vi "ADC Initiate Digitizing Process.vi"(8 "error in":errorcluster, 10 "Is first multiplex cycle? (True)":bool=TRUE, 11 "adc session in":T1={"niScope"={"channel cfg"=[], "sessions"=[], "multi cards"=FALSE, "channels"=0, "type"=enum."n/a", "memory [B/chn]"=0, "ext. clock [Hz]"=0.0, "samples count"=0, "use streaming"=FALSE, "proc setup"={"packet size [smpl]"=0, "current timeout [s]"=0.0, "blk2blk timeout [s]"=0.0, "event time"=timestamp(0 s since 1904-01-01), "temp sampl T [s]"=0.0, "data queue"=refnum, "stop notifier"=refnum, "proc ref"=refnum}, "sample width [B]"=0, "ranges [V]"=[], "trigger setup"={"coupling"=1, "level [V]"=0.0, "slope"=0, "mode"=enum."Immediate", "pre-trigger [%]"=0.0}, "fs [Hz]"=0.0, "bitres [bit]"=0, "clock source"=enum."VAL_NO_SOURCE"}, "3458A"={"channels"=[], "sync unit"={"VISA"="", "type"=enum."Picotest U6200A"}, "awg unit"={"type"=enum."Agilent 331xxA to 332xxA", "VISA"="", "enable 10MHz ref"=FALSE, "cmi ckd2"={"VISA"="", "clock source"=enum."Auto", "manual ref clk"=FALSE, "ref clock [Hz]"=0.0, "div mode"=enum."Set divisor directly"}, "cmi sync v3"={"VISA"="", "baud rate [bd/s]"=115200, "source"=enum."Auto", "hv range"=enum."1kV", "fsrc is fixed"=FALSE, "fsrc [Hz]"=10000000.0, "freq integ [s]"=1.0, "freq filter"=5, "trig level"=enum."TTL 5V", "chn1 mode"=enum."Source divider", "chn1 level"=enum."Positive 5V", "chn2 mode"=enum."Source divider", "chn2 level"=enum."Positive 5V", "chn2 div"=1, "chn3 mode"=enum."Chn 1 Active", "chn3 level"=enum."Positive 5V", "chn1 div entry"=enum."Calculate nearest divisor from measured fx", "chn1 dev limit [%]"=1.0, "chn1 check dev"=FALSE}, "trigger"={"source"=enum."Immediate", "slope"=enum."POS", "coupling"=enum."DC", "level [V]"=0.0, "hysteresis [V]"=0.0, "pre-trigger [%]"=0.0}, "HMF2500 cfg"={"Baud Rate"=9600, "Parity"=0, "Data Bits"=8, "Flow Control"=4}}, "sync mode"=enum."MASTER-SLAVE, MASTER clocked by TIMER", "streaming mode"=FALSE, "idn mode"=enum."Auto", "sampling mode"=enum."DCV", "sample memory [B]"=0, "proc setup"={"channel id"=0, "packet size [smpl]"=0, "current timeout [s]"=0.0, "blk2blk timeout [s]"=0.0, "event time"=timestamp(0 s since 1904-01-01), "stop notifier"=refnum, "data queues"=[], "proc refs"=[], "bus semaphore"=refnum}, "sample size [B]"=0, "sample count"=0, "aux data"={"channel id"=0, "valid?"=[], "gain [V]"=[], "timestamp [s]"=[], "Ts [s]"=0.0, "abs timestamp"=timestamp(0 s since 1904-01-01), "t [deg C]"=[], "multiplex timestamp [s]"=-1.0, "only multiplex?"=FALSE, "multiplex smpl offset"=0, "overflow?"=FALSE}, "ranges [V]"=[], "aperture [s]"=0.0, "LEVEL trigger"={"edge"=enum."POS", "level [V]"=0.0, "coupling"=enum."DC"}, "trigger mode"=enum."AUTO", "measure temp.?"=FALSE, "disp mesages"=[], "shared bus?"=FALSE, "disable display?"=FALSE, "aper mode"=enum."Manual", "aper rules"=[], "multiplex"={"cycles"=0, "delay [s]"=0.0, "enabled"=FALSE, "overhead [s]"=1.0, "tot smpls"=0, "sub-rec"=0, "overhead [%]"=0.0, "emulated"=FALSE}, "F8588 lpf"=enum."Off", "F8588 pll"=enum."Off", "F8588 couple"=enum."DC, auto", "fs"={"freq mode"=enum."fs or Ts", "fs [Hz]"=0.0, "fref [Hz]"=0.0, "mul"=0.0, "div"=0.0}, "fs mode"=enum."fs or Ts"}, "dsdll"={"dsdll"={"dsdll path"=path "", "dsdll handle"=[], "output devices"=[], "capture devices"=[]}, "channels"=0, "device id"=0, "channel idns"=[], "proc setup"={"packet size [smpl]"=0, "current timeout [s]"=0.0, "blk2blk timeout [s]"=0.0, "event time"=timestamp(0 s since 1904-01-01), "data queue"=refnum, "stop notifier"=refnum, "proc ref"=refnum}, "samples count"=0, "fs [Hz]"=0.0}, "type"=enum."niScope", "channel idn str"=[], "aux instr idn str"=[], "modified?"=FALSE, "simadc"={"channels"=[], "range [V]"=0.0, "Ts step [s]"=0.0, "time [s]"=0.0, "fs [Hz]"=0.0, "count"=0, "smpl offset"=0, "set count"=0, "bit res"=0}, "force rst?"=FALSE, "exit mode"=enum."Immediate reset", "exit dly"=0.0, "exit tmr"=timestamp(0 s since 1904-01-01), "busy?"=FALSE, "accessed?"=FALSE, "multiplex"={"Type"=enum."Dummy", "gen com ssn"={"visa"="", "primary"=enum."None", "secondary"=enum."None", "channels"=[]}, "delay before [s]"=0.0, "delay post [s]"=0.0, "sequence"=[], "enabled"=FALSE, "ref timestamp [s]"=0.0, "idn string"="", "dev niScope"="", "niScope idx"=0, "QPMX ssn"={"visa"="", "switch mode"=enum."Switched by TWM", "sequence"=[], "timing delays"=[], "polarity"=enum."Positive", "ss delay (s)"=2.0, "internal timer (s)"=1.0, "Last loaded sequence file"=path "", "startup delay (s)"=2.0}, "VISA mux ssn"={"VISA"="", "paths"=[], "idn command"="", "serial cfg"={"Baud rate"=9600, "Data bits"=8, "Parity"=0, "Stop bits"=10, "Flow control"=0, "End Mode Read"=enum."None", "End Mode Write"=enum."None", "Term character"=0, "Term enable"=FALSE}}}, "keysight dso"={"VISA"="", "channels"=[], "bw limit [Hz]"=0.0, "resolution"=enum."Basic", "trig noise reject"=enum."Normal", "N"=0, "trigger config"={"trigger source"=enum."Immediate", "trigger slope"=enum."Negative", "level [V]"=0.0, "hysteresis [V]"=0.001, "pre-trig [%]"=50}, "fs [Hz]"=0.0, "timeout stop"=timestamp(0 s since 1904-01-01), "waiting for opc"=FALSE, "fetch offset [smpl]"=0, "abs timestamp"=timestamp(0 s since 1904-01-01), "ranges [V]"=[], "decimation"=1.0, "ext ref"=FALSE, "emulate aperture"=FALSE, "model"=enum."DSO91304"}, "cdaq"={"mclk [Hz]"=12800000.0, "ADC task"="", "mclk reference"="", "fs [Hz]"=50000.0, "queue adc cmd"=refnum, "queue adc data"=refnum, "adc proc ref"=refnum, "channels"=[], "last channels"=[], "timeout"=timestamp(0 s since 1904-01-01), "N"=1000, "mclk mode"=enum."Free running", "ext mclk source"=""}, "ignore overload"=FALSE, "ADS127L21"={"VISA"="", "chn list"=[], "record size"=0, "phys. channels"=0, "adc fifo size"=0, "channels"=[], "ext refclk?"=FALSE, "fs [Hz]"=0.0, "ext refclk [Hz]"=0.0, "meas refclk [Hz]"=0.0, "EXTOUT mode"=enum."ADCCLK", "EXTOUT polarity"=enum."NORM", "EXTOUT divisor"=0}} {"ADS127L21"."channels"."Channel" min=1 max=8 step=1; "cdaq"."last channels"."Channel id" min=0 step=1; "cdaq"."channels"."Channel id" min=0 step=1; "keysight dso"."decimation" min=1.0; "keysight dso"."bw limit [Hz]" format="%#_6p"; "keysight dso"."channels"."Offset [V]" format="%#_6p"; "keysight dso"."channels"."Range [Vpk]" min=0.0 format="%#_6p"; "keysight dso"."channels"."Channel" min=1; "multiplex"."VISA mux ssn"."serial cfg"."Flow control" items=["None", "XON/XOFF", "CTS/RTS", "XON/XOFF + CTS/RTS", "DTR/DSR", "XON/XOFF + DTR/DSR"]; "multiplex"."VISA mux ssn"."serial cfg"."Stop bits" items=["1 bit"=10, "1.5 bits"=15, "2 bits"=20]; "multiplex"."VISA mux ssn"."serial cfg"."Parity" items=["None", "Odd", "Even", "Mark", "Space"]; "multiplex"."VISA mux ssn"."serial cfg"."Data bits" items=["5 bits"=5, "6 bits"=6, "7 bits"=7, "8 bits"=8]; "multiplex"."VISA mux ssn"."serial cfg"."Baud rate" items=["150 Bd"=150, "300 Bd"=300, "600 Bd"=600, "1200 Bd"=1200, "2400 Bd"=2400, "4800 Bd"=4800, "9600 Bd"=9600, "19.2 kBd"=19200, "38.4 kBd"=38400, "57.6 kBd"=57600, "115.2 kBd"=115200]; "multiplex"."QPMX ssn"."startup delay (s)" min=0.0 step=1.0; "multiplex"."QPMX ssn"."internal timer (s)" min=0.0 step=1.0; "multiplex"."QPMX ssn"."ss delay (s)" min=0.0 step=1.0; "multiplex"."QPMX ssn"."timing delays" min=1 max=255 step=1; "3458A"."awg unit"."HMF2500 cfg"."Flow Control" items=["None", "XON/XOFF", "RTS/CTS", "XON/XOFF & RTS/CTS", "DTR/DSR", "XON/XOFF & DTR/DSR"]; "3458A"."awg unit"."HMF2500 cfg"."Data Bits" items=["7"=7, "8"=8]; "3458A"."awg unit"."HMF2500 cfg"."Parity" items=["None", "Odd", "Even", "Mark", "Space"]; "3458A"."awg unit"."HMF2500 cfg"."Baud Rate" items=["300"=300, "600"=600, "1200"=1200, "2400"=2400, "4800"=4800, "9600"=9600, "19200"=19200]; "3458A"."awg unit"."cmi sync v3"."chn2 div" min=1 max=100000000 step=1; "3458A"."awg unit"."cmi sync v3"."fsrc [Hz]" format="%_8p"; "3458A"."channels"."Range [Vpk]" min=0.0; "niScope"."trigger setup"."pre-trigger [%]" format="%.2f"; "niScope"."trigger setup"."level [V]" format="%.2f"; "niScope"."trigger setup"."coupling" items=["AC"=0, "DC"=1, "HF Reject"=3, "LF Reject"=4, "AC Plus HF Reject"=1001]; "niScope"."channel cfg"."Range [Vpk]" min=0.0; "niScope"."channel cfg"."Channel" min=0}) -> (0 "error out":errorcluster, 3 "adc session out":T1={"niScope"={"channel cfg"=[], "sessions"=[], "multi cards"=FALSE, "channels"=0, "type"=enum."n/a", "memory [B/chn]"=0, "ext. clock [Hz]"=0.0, "samples count"=0, "use streaming"=FALSE, "proc setup"={"packet size [smpl]"=0, "current timeout [s]"=0.0, "blk2blk timeout [s]"=0.0, "event time"=timestamp(0 s since 1904-01-01), "temp sampl T [s]"=0.0, "data queue"=refnum, "stop notifier"=refnum, "proc ref"=refnum}, "sample width [B]"=0, "ranges [V]"=[], "trigger setup"={"coupling"=1, "level [V]"=0.0, "slope"=0, "mode"=enum."Immediate", "pre-trigger [%]"=0.0}, "fs [Hz]"=0.0, "bitres [bit]"=0, "clock source"=enum."VAL_NO_SOURCE"}, "3458A"={"channels"=[], "sync unit"={"VISA"="", "type"=enum."Picotest U6200A"}, "awg unit"={"type"=enum."Agilent 331xxA to 332xxA", "VISA"="", "enable 10MHz ref"=FALSE, "cmi ckd2"={"VISA"="", "clock source"=enum."Auto", "manual ref clk"=FALSE, "ref clock [Hz]"=0.0, "div mode"=enum."Set divisor directly"}, "cmi sync v3"={"VISA"="", "baud rate [bd/s]"=115200, "source"=enum."Auto", "hv range"=enum."1kV", "fsrc is fixed"=FALSE, "fsrc [Hz]"=10000000.0, "freq integ [s]"=1.0, "freq filter"=5, "trig level"=enum."TTL 5V", "chn1 mode"=enum."Source divider", "chn1 level"=enum."Positive 5V", "chn2 mode"=enum."Source divider", "chn2 level"=enum."Positive 5V", "chn2 div"=1, "chn3 mode"=enum."Chn 1 Active", "chn3 level"=enum."Positive 5V", "chn1 div entry"=enum."Calculate nearest divisor from measured fx", "chn1 dev limit [%]"=1.0, "chn1 check dev"=FALSE}, "trigger"={"source"=enum."Immediate", "slope"=enum."POS", "coupling"=enum."DC", "level [V]"=0.0, "hysteresis [V]"=0.0, "pre-trigger [%]"=0.0}, "HMF2500 cfg"={"Baud Rate"=9600, "Parity"=0, "Data Bits"=8, "Flow Control"=4}}, "sync mode"=enum."MASTER-SLAVE, MASTER clocked by TIMER", "streaming mode"=FALSE, "idn mode"=enum."Auto", "sampling mode"=enum."DCV", "sample memory [B]"=0, "proc setup"={"channel id"=0, "packet size [smpl]"=0, "current timeout [s]"=0.0, "blk2blk timeout [s]"=0.0, "event time"=timestamp(0 s since 1904-01-01), "stop notifier"=refnum, "data queues"=[], "proc refs"=[], "bus semaphore"=refnum}, "sample size [B]"=0, "sample count"=0, "aux data"={"channel id"=0, "valid?"=[], "gain [V]"=[], "timestamp [s]"=[], "Ts [s]"=0.0, "abs timestamp"=timestamp(0 s since 1904-01-01), "t [deg C]"=[], "multiplex timestamp [s]"=-1.0, "only multiplex?"=FALSE, "multiplex smpl offset"=0, "overflow?"=FALSE}, "ranges [V]"=[], "aperture [s]"=0.0, "LEVEL trigger"={"edge"=enum."POS", "level [V]"=0.0, "coupling"=enum."DC"}, "trigger mode"=enum."AUTO", "measure temp.?"=FALSE, "disp mesages"=[], "shared bus?"=FALSE, "disable display?"=FALSE, "aper mode"=enum."Manual", "aper rules"=[], "multiplex"={"cycles"=0, "delay [s]"=0.0, "enabled"=FALSE, "overhead [s]"=1.0, "tot smpls"=0, "sub-rec"=0, "overhead [%]"=0.0, "emulated"=FALSE}, "F8588 lpf"=enum."Off", "F8588 pll"=enum."Off", "F8588 couple"=enum."DC, auto", "fs"={"freq mode"=enum."fs or Ts", "fs [Hz]"=0.0, "fref [Hz]"=0.0, "mul"=0.0, "div"=0.0}, "fs mode"=enum."fs or Ts"}, "dsdll"={"dsdll"={"dsdll path"=path "", "dsdll handle"=[], "output devices"=[], "capture devices"=[]}, "channels"=0, "device id"=0, "channel idns"=[], "proc setup"={"packet size [smpl]"=0, "current timeout [s]"=0.0, "blk2blk timeout [s]"=0.0, "event time"=timestamp(0 s since 1904-01-01), "data queue"=refnum, "stop notifier"=refnum, "proc ref"=refnum}, "samples count"=0, "fs [Hz]"=0.0}, "type"=enum."niScope", "channel idn str"=[], "aux instr idn str"=[], "modified?"=FALSE, "simadc"={"channels"=[], "range [V]"=0.0, "Ts step [s]"=0.0, "time [s]"=0.0, "fs [Hz]"=0.0, "count"=0, "smpl offset"=0, "set count"=0, "bit res"=0}, "force rst?"=FALSE, "exit mode"=enum."Immediate reset", "exit dly"=0.0, "exit tmr"=timestamp(0 s since 1904-01-01), "busy?"=FALSE, "accessed?"=FALSE, "multiplex"={"Type"=enum."Dummy", "gen com ssn"={"visa"="", "primary"=enum."None", "secondary"=enum."None", "channels"=[]}, "delay before [s]"=0.0, "delay post [s]"=0.0, "sequence"=[], "enabled"=FALSE, "ref timestamp [s]"=0.0, "idn string"="", "dev niScope"="", "niScope idx"=0, "QPMX ssn"={"visa"="", "switch mode"=enum."Switched by TWM", "sequence"=[], "timing delays"=[], "polarity"=enum."Positive", "ss delay (s)"=2.0, "internal timer (s)"=1.0, "Last loaded sequence file"=path "", "startup delay (s)"=2.0}, "VISA mux ssn"={"VISA"="", "paths"=[], "idn command"="", "serial cfg"={"Baud rate"=9600, "Data bits"=8, "Parity"=0, "Stop bits"=10, "Flow control"=0, "End Mode Read"=enum."None", "End Mode Write"=enum."None", "Term character"=0, "Term enable"=FALSE}}}, "keysight dso"={"VISA"="", "channels"=[], "bw limit [Hz]"=0.0, "resolution"=enum."Basic", "trig noise reject"=enum."Normal", "N"=0, "trigger config"={"trigger source"=enum."Immediate", "trigger slope"=enum."Negative", "level [V]"=0.0, "hysteresis [V]"=0.001, "pre-trig [%]"=50}, "fs [Hz]"=0.0, "timeout stop"=timestamp(0 s since 1904-01-01), "waiting for opc"=FALSE, "fetch offset [smpl]"=0, "abs timestamp"=timestamp(0 s since 1904-01-01), "ranges [V]"=[], "decimation"=1.0, "ext ref"=FALSE, "emulate aperture"=FALSE, "model"=enum."DSO91304"}, "cdaq"={"mclk [Hz]"=12800000.0, "ADC task"="", "mclk reference"="", "fs [Hz]"=50000.0, "queue adc cmd"=refnum, "queue adc data"=refnum, "adc proc ref"=refnum, "channels"=[], "last channels"=[], "timeout"=timestamp(0 s since 1904-01-01), "N"=1000, "mclk mode"=enum."Free running", "ext mclk source"=""}, "ignore overload"=FALSE, "ADS127L21"={"VISA"="", "chn list"=[], "record size"=0, "phys. channels"=0, "adc fifo size"=0, "channels"=[], "ext refclk?"=FALSE, "fs [Hz]"=0.0, "ext refclk [Hz]"=0.0, "meas refclk [Hz]"=0.0, "EXTOUT mode"=enum."ADCCLK", "EXTOUT polarity"=enum."NORM", "EXTOUT divisor"=0}} {"ADS127L21"."channels"."Channel" min=1 max=8 step=1; "cdaq"."last channels"."Channel id" min=0 step=1; "cdaq"."channels"."Channel id" min=0 step=1; "keysight dso"."decimation" min=1.0; "keysight dso"."bw limit [Hz]" format="%#_6p"; "keysight dso"."channels"."Offset [V]" format="%#_6p"; "keysight dso"."channels"."Range [Vpk]" min=0.0 format="%#_6p"; "keysight dso"."channels"."Channel" min=1; "multiplex"."VISA mux ssn"."serial cfg"."Flow control" items=["None", "XON/XOFF", "CTS/RTS", "XON/XOFF + CTS/RTS", "DTR/DSR", "XON/XOFF + DTR/DSR"]; "multiplex"."VISA mux ssn"."serial cfg"."Stop bits" items=["1 bit"=10, "1.5 bits"=15, "2 bits"=20]; "multiplex"."VISA mux ssn"."serial cfg"."Parity" items=["None", "Odd", "Even", "Mark", "Space"]; "multiplex"."VISA mux ssn"."serial cfg"."Data bits" items=["5 bits"=5, "6 bits"=6, "7 bits"=7, "8 bits"=8]; "multiplex"."VISA mux ssn"."serial cfg"."Baud rate" items=["150 Bd"=150, "300 Bd"=300, "600 Bd"=600, "1200 Bd"=1200, "2400 Bd"=2400, "4800 Bd"=4800, "9600 Bd"=9600, "19.2 kBd"=19200, "38.4 kBd"=38400, "57.6 kBd"=57600, "115.2 kBd"=115200]; "multiplex"."QPMX ssn"."startup delay (s)" min=0.0 step=1.0; "multiplex"."QPMX ssn"."internal timer (s)" min=0.0 step=1.0; "multiplex"."QPMX ssn"."ss delay (s)" min=0.0 step=1.0; "multiplex"."QPMX ssn"."timing delays" min=1 max=255 step=1; "3458A"."awg unit"."HMF2500 cfg"."Flow Control" items=["None", "XON/XOFF", "RTS/CTS", "XON/XOFF & RTS/CTS", "DTR/DSR", "XON/XOFF & DTR/DSR"]; "3458A"."awg unit"."HMF2500 cfg"."Data Bits" items=["7"=7, "8"=8]; "3458A"."awg unit"."HMF2500 cfg"."Parity" items=["None", "Odd", "Even", "Mark", "Space"]; "3458A"."awg unit"."HMF2500 cfg"."Baud Rate" items=["300"=300, "600"=600, "1200"=1200, "2400"=2400, "4800"=4800, "9600"=9600, "19200"=19200]; "3458A"."awg unit"."cmi sync v3"."chn2 div" min=1 max=100000000 step=1; "3458A"."awg unit"."cmi sync v3"."fsrc [Hz]" format="%_8p"; "3458A"."channels"."Range [Vpk]" min=0.0; "niScope"."trigger setup"."pre-trigger [%]" format="%.2f"; "niScope"."trigger setup"."level [V]" format="%.2f"; "niScope"."trigger setup"."coupling" items=["AC"=0, "DC"=1, "HF Reject"=3, "LF Reject"=4, "AC Plus HF Reject"=1001]; "niScope"."channel cfg"."Range [Vpk]" min=0.0; "niScope"."channel cfg"."Channel" min=0})   [LabVIEW 2020]
doc: "Initiates digitizing process. It starts background processes that starts sampling as soon as trigger condition it meet. Then they either stores samples to the instruments memory and reading them afterwards or streams the data directly. In both cases the sample data are sent to data queue(s). The content of the queue must be read and processed as fast as possible to prevent overflow error so this VI call must be immediatelly followed by fetch loop with 'Fetch From Digitizing Process' function. When fetching is done for whatever reason user must call 'Clenup Digitizing Process' to kill and cleanup all objects related to the digitizing process. It must be called even in case of error.\nVI modifies session content so do not assign just ADC session in!\n\nInput 'Is first multiplex cycle?' must be True for first multiplexing cycle within the multiplexing sequence. For non-multiplex mode its value must be True (default)."
uses:
  ADC Session.ctl
  drivers/niScope/niScope Session.ctl
  drivers/niScope/niScope Virtual Channel Config.ctl
  drivers/niScope/niScope Virtual Channel Mode.ctl
  drivers/niScope/niScope Virtual Channel Input Z.ctl
  drivers/niScope/niScope Virtual Channel Coupling.ctl
  drivers/niScope/niScope Type.ctl
  drivers/niScope/niScope Digitizing Process Options.ctl
  drivers/niScope/niScope Data Packet.ctl
  drivers/niScope/niScope Trigger Setup.ctl
  <instrlib>/niScope/Controls/niScope trigger coupling.ctl
  <instrlib>/niScope/Controls/niScope trigger slope.ctl
  drivers/niScope/niScope Reference Clock.ctl
  drivers/DMM/3458A Digitizer Session.ctl
  drivers/DMM/3458A Virtual Channel Config.ctl
  drivers/Counter/Counter Session.ctl
  drivers/Counter/Counter Type.ctl
  drivers/AWG/AWG Session.ctl
  drivers/AWG/AWG Type.ctl
  drivers/AWG/CMI Clock Divider v2/CMI ckd2 Session.ctl
  drivers/AWG/CMI Clock Divider v2/CMI ckd2 Source Mode.ctl
  drivers/AWG/CMI Clock Divider v2/CMI ckd2 Divisor Mode.ctl
  drivers/AWG/CMI Sync V3/CMI Sync V3 session.ctl
  drivers/AWG/CMI Sync V3/Configure/CMI Sync V3 Reference Clock Source.ctl
  drivers/AWG/CMI Sync V3/Configure/CMI Sync V3 HV input Range.ctl
  drivers/AWG/CMI Sync V3/Configure/CMI Sync V3 Trigger Input Level.ctl
  drivers/AWG/CMI Sync V3/Configure/CMI Sync V3 Channel 1 Mode.ctl
  drivers/AWG/CMI Sync V3/Configure/CMI Sync V3 Channel Output Levels.ctl
  drivers/AWG/CMI Sync V3/Configure/CMI Sync V3 Channel 2 Mode.ctl
  drivers/AWG/CMI Sync V3/Configure/CMI Sync V3 Channel 3 Mode.ctl
  drivers/AWG/CMI Sync V3/Configure/CMI Sync V3 Channel 1 Divisor Entry Mode.ctl
  ADC Trig Config.ctl
  ADC Trig Mode Source.ctl
  ADC Trig Slope.ctl
  ADC Trig Coupling.ctl
  drivers/AWG/RaS HMF2500/HMF2500 Config.ctl
  drivers/DMM/3458A Sync Mode.ctl
  drivers/DMM/3458A Idn Mode.ctl
  drivers/DMM/3458A Digitizing Low Levels/Configure/Sampling Mode.ctl
  drivers/DMM/3458A Digitizing Process Options.ctl
  drivers/DMM/3458A Data Packet.ctl
  drivers/DMM/3458A Aux Record Data.ctl
  drivers/DMM/3458A Digitizing Low Levels/Configure/Level Setup.ctl
  drivers/DMM/3458A Digitizing Low Levels/Configure/First Sample Trigger.ctl
  drivers/DMM/3458A Aperture Selection Mode.ctl
  drivers/DMM/3458A Multiplexing Config.ctl
  drivers/Fluke 8588A/F8588A Low Pass Filter.ctl
  drivers/Fluke 8588A/F8588A Phase Lock.ctl
  drivers/Fluke 8588A/F8588A Coupling.ctl
  drivers/DMM/3458A Sampling Rate.ctl
  drivers/AWG/AWG Clock Setup Mode.ctl
  drivers/DMM/3458A Sample Rate Mode.ctl
  drivers/dsdll/DSDLL Session.ctl
  drivers/dsdll/dsdll/dsdll_instance.ctl
  drivers/dsdll/dsdll/dsdll_device_record.ctl
  drivers/dsdll/DSDLL Process Config.ctl
  drivers/dsdll/DSDLL Data Packet.ctl
  ADC Type.ctl
  drivers/simulated_adc/SimAdc Config.ctl
  drivers/simulated_adc/SimAdc Channel Cfg.ctl
  ADC On Close Action.ctl
  Multiplexer/MPX Session.ctl
  Multiplexer/MPX Type.ctl
  drivers/Multiplexers/Generic COM/GCOMM Session.ctl
  drivers/Multiplexers/Generic COM/GCOMM Signal.ctl
  drivers/Multiplexers/Generic COM/GCOMM Virtual Channel.ctl
  drivers/Multiplexers/Generic COM/GCOMM Logic State.ctl
  drivers/Multiplexers/Generic COM/QPMX Session.ctl
  drivers/Multiplexers/QPMX/QPMX switch mode.ctl
  drivers/Multiplexers/QPMX/QPMX polarity.ctl
  drivers/Multiplexers/Generic VISA commands/GVISA Mux Session.ctl
  drivers/Multiplexers/Generic VISA commands/GVISA Mux Path Entry.ctl
  drivers/Multiplexers/Generic VISA commands/met_serial_setup.ctl
  drivers/Agilent DSO 90000/Virtual Digitizer/KeDSO session.ctl
  drivers/Agilent DSO 90000/Virtual Digitizer/KeDSO Virtual Channel.ctl
  drivers/Agilent DSO 90000/Virtual Digitizer/KeDSO High Resolution Mode.ctl
  drivers/Agilent DSO 90000/Virtual Digitizer/KeDSO Trigger Setup.ctl
  drivers/Agilent DSO 90000/Virtual Digitizer/KeDSO Trigger Source.ctl
  drivers/Agilent DSO 90000/Public/Utility/DSO type.ctl
  drivers/cdaq/cDAQ Session.ctl
  drivers/cdaq/low_level_old/cdaq_anal_adc_command.ctl
  drivers/cdaq/low_level_old/cdaq_anal_adc_data.ctl
  drivers/cdaq/cDAQ Virtual Channel.ctl
  drivers/cdaq/cDAQ Master Clock Mode.ctl
  drivers/CMI_ADS127L21/CMI ADS127L21 - Session.ctl
  drivers/CMI_ADS127L21/CMI ADS127L21 - Record Channel.ctl
  drivers/CMI_ADS127L21/CMI ADS127L21 - Input Range.ctl
  drivers/CMI_ADS127L21/CMI ADS127L21 - Input Mode.ctl
  drivers/CMI_ADS127L21/CMI ADS127L21 - Input Impedance.ctl
  drivers/CMI_ADS127L21/CMI ADS127L21 - EXTOUT Mode.ctl
  drivers/CMI_ADS127L21/CMI ADS127L21 - EXTOUT Polarity.ctl
  drivers/niScope/niScope Virtual Digitizer.lvlib
  drivers/DMM/3458A Virtual Digitizer.lvlib
  drivers/dsdll/DSDLL Virtual Digitizer.lvlib
  <vilib>/Utility/error.llb/Error Cluster From Error Code.vi
  <vilib>/ErrorRing/Error Ring.xnode
  drivers/Counter/Counter.lvlib
  drivers/AWG/AWG.lvlib
  drivers/DMM/3458A Digitizing Low Levels/3458A Digitizing Low Levels.lvlib
  drivers/dsdll/dsdll/dsdll.lvlib
  drivers/AWG/CMI Sync V3/CMI Sync Unit V3.lvlib
  drivers/Agilent DSO 90000/Agilent 90000 Series.lvlib
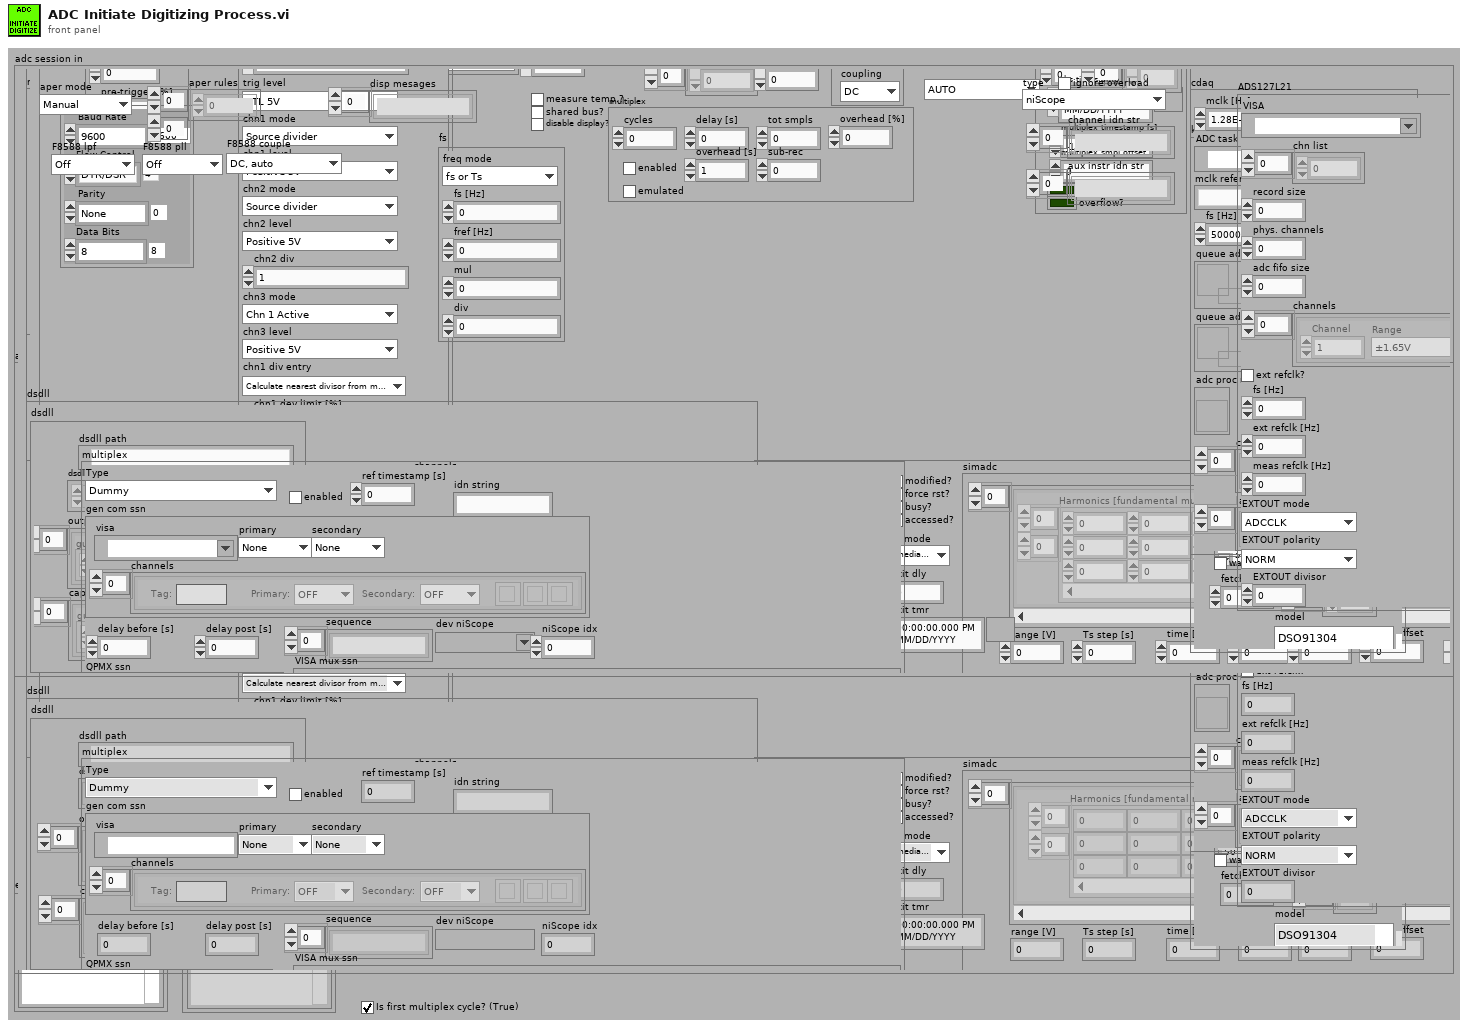
[diagram p1: front panel]
types:
  T1 = typedef "ADC Session.ctl" = cluster{"niScope":T2, "3458A":T13, "dsdll":T52, "type":T56, "channel idn str":string[], "aux instr idn str":string[], "modified?":bool, "simadc":T57, "force rst?":bool, "exit mode":T59, "exit dly":dbl, "exit tmr":timestamp, "busy?":bool, "accessed?":bool, "multiplex":T60, "keysight dso":T72, "cdaq":T78, "ignore overload":bool, "ADS127L21":T81}
  T2 = typedef "niScope Virtual Digitizer.lvlib/niScope Session.ctl" = cluster{"channel cfg":T3[], "sessions":refnum<k20>[], "multi cards":bool, "channels":i32, "type":T7, "memory [B/chn]":i32, "ext. clock [Hz]":dbl, "samples count":i64, "use streaming":bool, "proc setup":T8, "sample width [B]":i32, "ranges [V]":dbl[], "trigger setup":T9, "fs [Hz]":dbl, "bitres [bit]":i32, "clock source":T12}
  T3 = typedef "niScope Virtual Digitizer.lvlib/niScope Virtual Channel Config.ctl" = cluster{"Address":refnum<k15>, "Channel":i32, "Mode":T4, "Input Z":T5, "Coupling":T6, "Range [Vpk]":dbl, "btn clr":bool, "btn up":bool, "btn down":bool}
  T4 = typedef "niScope Virtual Digitizer.lvlib/niScope Virtual Channel Mode.ctl" = enum16{"Single ended", "Unbal. differential", "Differential"}
  T5 = typedef "niScope Virtual Digitizer.lvlib/niScope Virtual Channel Input Z.ctl" = enum16{"1 MOhm", "50 Ohm"}
  T6 = typedef "niScope Virtual Digitizer.lvlib/niScope Virtual Channel Coupling.ctl" = enum16{"AC", "DC", "GND"}
  T7 = typedef "niScope Virtual Digitizer.lvlib/niScope Type.ctl" = enum16{"n/a", "5922"}
  T8 = typedef "niScope Virtual Digitizer.lvlib/niScope Digitizing Process Options.ctl" = cluster{"packet size [smpl]":i64, "current timeout [s]":dbl, "blk2blk timeout [s]":dbl, "event time":timestamp, "temp sampl T [s]":dbl, "data queue":refnum<queue>, "stop notifier":refnum<notifier>, "proc ref":refnum<vi>}
  T9 = typedef "niScope Virtual Digitizer.lvlib/niScope Trigger Setup.ctl" = cluster{"coupling":T10, "level [V]":dbl, "slope":T11, "mode":enum16{"Immediate", "External", "Level"}, "pre-trigger [%]":dbl}
  T10 = typedef "niScope trigger coupling.ctl" = u16
  T11 = typedef "niScope trigger slope.ctl" = i32
  T12 = typedef "niScope Virtual Digitizer.lvlib/niScope Reference Clock.ctl" = enum16{"VAL_NO_SOURCE", "VAL_CLK_IN", "VAL_PXI_CLOCK", "VAL_EXTERNAL"}
  T13 = typedef "3458A Virtual Digitizer.lvlib/3458A Digitizer Session.ctl" = cluster{"channels":T14[], "sync unit":T15, "awg unit":T17, "sync mode":T36, "streaming mode":bool, "idn mode":T37, "sampling mode":T38, "sample memory [B]":i32, "proc setup":T39, "sample size [B]":i32, "sample count":i32, "aux data":T41, "ranges [V]":dbl[], "aperture [s]":dbl, "LEVEL trigger":T42, "trigger mode":T43, "measure temp.?":bool, "disp mesages":string[], "shared bus?":bool, "disable display?":bool, "aper mode":T44, "aper rules":dbl[][], "multiplex":T45, "F8588 lpf":T46, "F8588 pll":T47, "F8588 couple":T48, "fs":T49, "fs mode":T51}
  T14 = typedef "3458A Virtual Digitizer.lvlib/3458A Virtual Channel Config.ctl" = cluster{"VISA":refnum<visa-resource-name>, "Range [Vpk]":dbl, "btn clr":bool, "btn up":bool, "btn down":bool, "F8588":bool, "F8588 guard":bool}
  T15 = typedef "Counter.lvlib/Counter Session.ctl" = cluster{"VISA":refnum<visa-resource-name>, "type":T16}
  T16 = typedef "Counter.lvlib/Counter Type.ctl" = enum16{"Picotest U6200A", "dummy"}
  T17 = typedef "AWG.lvlib/AWG Session.ctl" = cluster{"type":T18, "VISA":refnum<visa-resource-name>, "enable 10MHz ref":bool, "cmi ckd2":T19, "cmi sync v3":T22, "trigger":T31, "HMF2500 cfg":T35}
  T18 = typedef "AWG.lvlib/AWG Type.ctl" = enum16{"Agilent 331xxA to 332xxA", "Agilent 335xxA to 336xxA", "Tektronix AFG3101C", "R&S HMF25xx", "CMI Clock Divider v2", "CMI Sync Unit V3", "dummy"}
  T19 = typedef "AWG.lvlib/CMI ckd2 Session.ctl" = cluster{"VISA":refnum<visa-resource-name>, "clock source":T20, "manual ref clk":bool, "ref clock [Hz]":dbl, "div mode":T21}
  T20 = typedef "AWG.lvlib/CMI ckd2 Source Mode.ctl" = enum16{"Auto", "LF clock", "HF clock", "Internal"}
  T21 = typedef "AWG.lvlib/CMI ckd2 Divisor Mode.ctl" = enum16{"Set divisor directly", "Set divisor by frequency"}
  T22 = typedef "AWG.lvlib/CMI Sync Unit V3.lvlib/CMI Sync V3 session.ctl" = cluster{"VISA":refnum<visa-resource-name>, "baud rate [bd/s]":i32, "source":T23, "hv range":T24, "fsrc is fixed":bool, "fsrc [Hz]":dbl, "freq integ [s]":dbl, "freq filter":i32, "trig level":T25, "chn1 mode":T26, "chn1 level":T27, "chn2 mode":T28, "chn2 level":T27, "chn2 div":i32, "chn3 mode":T29, "chn3 level":T27, "chn1 div entry":T30, "chn1 dev limit [%]":dbl, "chn1 check dev":bool}
  T23 = typedef "AWG.lvlib/CMI Sync Unit V3.lvlib/CMI Sync V3 Reference Clock Source.ctl" = enum16{"Auto", "Internal", "Logic", "Sine", "HV"}
  T24 = typedef "AWG.lvlib/CMI Sync Unit V3.lvlib/CMI Sync V3 HV input Range.ctl" = enum16{"10V", "60V", "250V", "1kV"}
  T25 = typedef "AWG.lvlib/CMI Sync Unit V3.lvlib/CMI Sync V3 Trigger Input Level.ctl" = enum16{"LVCMOS 3V3", "TTL 5V"}
  T26 = typedef "AWG.lvlib/CMI Sync Unit V3.lvlib/CMI Sync V3 Channel 1 Mode.ctl" = enum16{"Source divider", "DDS absolute", "DDS ratio", "DDS ratio M/N"}
  T27 = typedef "AWG.lvlib/CMI Sync Unit V3.lvlib/CMI Sync V3 Channel Output Levels.ctl" = enum16{"Positive 3V3", "Negative 3V3", "Positive 5V", "Negative 5V"}
  T28 = typedef "AWG.lvlib/CMI Sync Unit V3.lvlib/CMI Sync V3 Channel 2 Mode.ctl" = enum16{"Source divider", "Chn 1 divide"}
  T29 = typedef "AWG.lvlib/CMI Sync Unit V3.lvlib/CMI Sync V3 Channel 3 Mode.ctl" = enum16{"Chn 1 Active", "Chn 2 Active", "Chn 1 Trigger", "Chn 2 Trigger", "Gate", "PPS", "10MHz"}
  T30 = typedef "AWG.lvlib/CMI Sync Unit V3.lvlib/CMI Sync V3 Channel 1 Divisor Entry Mode.ctl" = enum16{"Set divisor directly", "Calculate nearest divisor from measured fx"}
  T31 = typedef "ADC Trig Config.ctl" = cluster{"source":T32, "slope":T33, "coupling":T34, "level [V]":dbl, "hysteresis [V]":dbl, "pre-trigger [%]":dbl}
  T32 = typedef "ADC Trig Mode Source.ctl" = enum16{"Immediate", "External", "Level"}
  T33 = typedef "ADC Trig Slope.ctl" = enum16{"POS", "NEG"}
  T34 = typedef "ADC Trig Coupling.ctl" = enum16{"DC", "AC"}
  T35 = typedef "AWG.lvlib/HMF2500 Config.ctl" = cluster{"Baud Rate":u32, "Parity":u16, "Data Bits":u16, "Flow Control":u16}
  T36 = typedef "3458A Virtual Digitizer.lvlib/3458A Sync Mode.ctl" = enum16{"MASTER-SLAVE, MASTER clocked by TIMER", "MASTER-SLAVE, MASTER clocked by AWG", "ALL clocked by AWG", "MASTER-SLAVE, ALL clocked by TIMER", "ALL clocked by AWG with DFLL"}
  T37 = typedef "3458A Virtual Digitizer.lvlib/3458A Idn Mode.ctl" = enum16{"Auto", "Sequential (chn A, chn B, ...)", "From calibration string"}
  T38 = typedef "3458A Virtual Digitizer.lvlib/3458A Digitizing Low Levels.lvlib/Sampling Mode.ctl" = enum16{"DCV", "DSDC", "DSAC"}
  T39 = typedef "3458A Virtual Digitizer.lvlib/3458A Digitizing Process Options.ctl" = cluster{"channel id":i32, "packet size [smpl]":i32, "current timeout [s]":dbl, "blk2blk timeout [s]":dbl, "event time":timestamp, "stop notifier":refnum<notifier>, "data queues":refnum<queue>[], "proc refs":refnum<vi>[], "bus semaphore":T40}
  T40 = typedef "Semaphore RefNum" = refnum<k1>
  T41 = typedef "3458A Virtual Digitizer.lvlib/3458A Aux Record Data.ctl" = cluster{"channel id":i32, "valid?":bool[], "gain [V]":dbl[], "timestamp [s]":dbl[], "Ts [s]":dbl, "abs timestamp":timestamp, "t [deg C]":dbl[], "multiplex timestamp [s]":dbl, "only multiplex?":bool, "multiplex smpl offset":i64, "overflow?":bool}
  T42 = typedef "3458A Virtual Digitizer.lvlib/3458A Digitizing Low Levels.lvlib/Level Setup.ctl" = cluster{"edge":enum16{"POS", "NEG"}, "level [V]":dbl, "coupling":enum16{"DC", "AC"}}
  T43 = typedef "3458A Virtual Digitizer.lvlib/3458A Digitizing Low Levels.lvlib/First Sample Trigger.ctl" = enum16{"AUTO", "EXT", "SYN", "SGL", "HOLD", "LEVEL"}
  T44 = typedef "3458A Virtual Digitizer.lvlib/3458A Aperture Selection Mode.ctl" = enum16{"Manual", "Maximum", "Table"}
  T45 = typedef "3458A Virtual Digitizer.lvlib/3458A Multiplexing Config.ctl" = cluster{"cycles":i32, "delay [s]":dbl, "enabled":bool, "overhead [s]":dbl, "tot smpls":i64, "sub-rec":i32, "overhead [%]":dbl, "emulated":bool}
  T46 = typedef "F8588A Low Pass Filter.ctl" = enum16{"Off", "100 kHz", "3 MHz"}
  T47 = typedef "F8588A Phase Lock.ctl" = enum16{"Off", "1 MHz", "10 MHz"}
  T48 = typedef "F8588A Coupling.ctl" = enum16{"AC, 1 MOhm", "AC, 10 MOhm", "DC, 1 MOhm", "DC, 10 MOhm", "DC, auto"}
  T49 = typedef "3458A Virtual Digitizer.lvlib/3458A Sampling Rate.ctl" = cluster{"freq mode":T50, "fs [Hz]":dbl, "fref [Hz]":dbl, "mul":dbl, "div":dbl}
  T50 = typedef "AWG.lvlib/AWG Clock Setup Mode.ctl" = enum16{"fs or Ts", "fs or Ts with fref", "fref/N", "fref*M/N", "fref*Ratio"}
  T51 = typedef "3458A Sample Rate Mode.ctl" = enum16{"fs or Ts", "fs*M/N"}
  T52 = typedef "DSDLL Virtual Digitizer.lvlib/DSDLL Session.ctl" = cluster{"dsdll":T53, "channels":i32, "device id":i32, "channel idns":string[], "proc setup":T55, "samples count":i32, "fs [Hz]":dbl}
  T53 = typedef "dsdll.lvlib/dsdll_instance.ctl" = cluster{"dsdll path":path, "dsdll handle":u8[], "output devices":T54[], "capture devices":T54[]}
  T54 = typedef "dsdll.lvlib/dsdll_device_record.ctl" = cluster{"guid":u8[], "name":string}
  T55 = typedef "DSDLL Virtual Digitizer.lvlib/DSDLL Process Config.ctl" = cluster{"packet size [smpl]":i32, "current timeout [s]":dbl, "blk2blk timeout [s]":dbl, "event time":timestamp, "data queue":refnum<queue>, "stop notifier":refnum<notifier>, "proc ref":refnum<vi>}
  T56 = typedef "ADC Type.ctl" = enum16{"niScope", "3458A", "DirectSound DLL", "Keysight DSO", "cDAQ ADC", "CMI ADS127L21", "dummy"}
  T57 = typedef "SimAdc Config.ctl" = cluster{"channels":T58[], "range [V]":dbl, "Ts step [s]":dbl, "time [s]":dbl, "fs [Hz]":dbl, "count":i64, "smpl offset":i64, "set count":i64, "bit res":i32}
  T58 = typedef "SimAdc Channel Cfg.ctl" = cluster{"harmonics":dbl[][], "btn clear":bool, "noise":dbl, "fundamental [Hz]":dbl}
  T59 = typedef "ADC On Close Action.ctl" = enum16{"Immediate reset", "Delayed reset"}
  T60 = typedef "MPX Session.ctl" = cluster{"Type":T61, "gen com ssn":T62, "delay before [s]":dbl, "delay post [s]":dbl, "sequence":string[], "enabled":bool, "ref timestamp [s]":dbl, "idn string":string, "dev niScope":refnum<k15>, "niScope idx":i32, "QPMX ssn":T66, "VISA mux ssn":T69}
  T61 = typedef "MPX Type.ctl" = enum16{"Dummy", "Generic - COM port", "Generic - niScope PFI", "Generic - VISA commands", "QPMX"}
  T62 = typedef "GCOMM Session.ctl" = cluster{"visa":refnum<visa-resource-name>, "primary":T63, "secondary":T63, "channels":T64[]}
  T63 = typedef "GCOMM Signal.ctl" = enum16{"None", "DTR", "RTS"}
  T64 = typedef "GCOMM Virtual Channel.ctl" = cluster{"Primary:":T65, "Secondary:":T65, "btn clr":bool, "btn up":bool, "btn down":bool, "Tag:":string}
  T65 = typedef "GCOMM Logic State.ctl" = enum16{"OFF", "ON"}
  T66 = typedef "QPMX Session.ctl" = cluster{"visa":refnum<visa-resource-name>, "switch mode":T67, "sequence":bool[][], "timing delays":u32[], "polarity":T68, "ss delay (s)":dbl, "internal timer (s)":dbl, "Last loaded sequence file":path, "startup delay (s)":dbl}
  T67 = typedef "QPMX switch mode.ctl" = enum16{"Switched by TWM", "Switched by external clock", "Switched by internal clock"}
  T68 = typedef "QPMX polarity.ctl" = enum16{"Positive", "Negative"}
  T69 = typedef "GVISA Mux Session.ctl" = cluster{"VISA":refnum<visa-resource-name>, "paths":T70[], "idn command":string, "serial cfg":T71}
  T70 = typedef "GVISA Mux Path Entry.ctl" = cluster{"Tag:":string, "Command:":string, "btn clr":bool, "btn up":bool, "btn down":bool}
  T71 = typedef "met_serial_setup.ctl" = cluster{"Baud rate":i32, "Data bits":i32, "Parity":i32, "Stop bits":i32, "Flow control":i32, "End Mode Read":enum16{"None", "Last Bit", "TermChar"}, "End Mode Write":enum16{"None", "Last Bit", "TermChar"}, "Term character":u8, "Term enable":bool}
  T72 = typedef "KeDSO session.ctl" = cluster{"VISA":refnum<visa-resource-name>, "channels":T73[], "bw limit [Hz]":dbl, "resolution":T74, "trig noise reject":enum16{"Normal", "High Sensitivity"}, "N":i64, "trigger config":T75, "fs [Hz]":dbl, "timeout stop":timestamp, "waiting for opc":bool, "fetch offset [smpl]":i64, "abs timestamp":timestamp, "ranges [V]":dbl[], "decimation":dbl, "ext ref":bool, "emulate aperture":bool, "model":T77}
  T73 = typedef "KeDSO Virtual Channel.ctl" = cluster{"Channel":i32, "Range [Vpk]":dbl, "btn clr":bool, "btn up":bool, "btn down":bool, "Offset [V]":dbl, "Coupling":enum16{"DC", "DC50", "AC", "LFR1"}, "bw limit enab":bool}
  T74 = typedef "KeDSO High Resolution Mode.ctl" = enum16{"Basic", "High-res AUTO", "Min. 9-bits", "Min. 10-bits", "Min. 11-bits", "Min. 12-bits", "Fixed 11-bits", "Fixed 12-bits", "Fixed 13-bits", "Fixed 14-bits", "Fixed 15-bits", "Fixed 16-bits"}
  T75 = typedef "KeDSO Trigger Setup.ctl" = cluster{"trigger source":T76, "trigger slope":enum16{"Negative", "Positive", "Either"}, "level [V]":dbl, "hysteresis [V]":dbl, "pre-trig [%]":i32}
  T76 = typedef "KeDSO Trigger Source.ctl" = enum16{"Immediate", "Level", "AUX"}
  T77 = typedef "Agilent 90000 Series.lvlib/DSO type.ctl" = enum16{"DSO91304", "DSO91204", "DSO90804", "DSO90604", "DSO90404", "DSO90254", "DSA91304", "DSA91204", "DSA90804", "DSA90604", "DSA90404", "DSA90254", "DSO9104", "DSO9254", "DSO9404", "MSO9104", "MSO9254", "MSO9404", "MSO9064", "DSO9064", "DSOX91604", "DSOX92004", "DSOX92504", "DSOX92804", "DSOX93204", "DSO93004", "DSO9024H", "DSO9054H", "DSO9104H", "DSO9204H", "DSOS054A", "DSOS104A", "DSOS204A", "DSOS254A", "DSOS404A", "DSOS604A", "DSOS804A", "MSOS054A", "MSOS104A", "MSOS204A", "MSOS254A", "MSOS404A", "MSOS604A", "MSOS804A", "DSAX96204Q", "DSOX96204Q", "DSAX95004Q", "DSOX95004Q", "DSAX93304Q", "DSOX93304Q", "DSAX92504Q", "DSOX92504Q", "DSAX92004Q", "DSOX92004Q"}
  T78 = typedef "cDAQ Session.ctl" = cluster{"mclk [Hz]":dbl, "ADC task":refnum<k21>, "mclk reference":string, "fs [Hz]":dbl, "queue adc cmd":refnum<queue>, "queue adc data":refnum<queue>, "adc proc ref":refnum<vi>, "channels":T79[], "last channels":T79[], "timeout":timestamp, "N":i32, "mclk mode":T80, "ext mclk source":tag}
  T79 = typedef "cDAQ Virtual Channel.ctl" = cluster{"Device":tag, "Channel id":i32, "btn clr":bool, "btn up":bool, "btn down":bool}
  T80 = typedef "cDAQ Master Clock Mode.ctl" = enum16{"Free running", "Export master clock", "Import master clock"}
  T81 = typedef "CMI ADS127L21 - Session.ctl" = cluster{"VISA":refnum<visa-resource-name>, "chn list":i32[], "record size":i32, "phys. channels":i32, "adc fifo size":i32, "channels":T82[], "ext refclk?":bool, "fs [Hz]":dbl, "ext refclk [Hz]":dbl, "meas refclk [Hz]":dbl, "EXTOUT mode":T86, "EXTOUT polarity":T87, "EXTOUT divisor":i32}
  T82 = typedef "CMI ADS127L21 - Record Channel.ctl" = cluster{"Range":T83, "Channel":i32, "Mode":T84, "Impedance":T85, "btn clr":bool, "btn up":bool, "btn down":bool}
  T83 = typedef "CMI ADS127L21 - Input Range.ctl" = enum16{"±1.65V", "±2V"}
  T84 = typedef "CMI ADS127L21 - Input Mode.ctl" = enum16{"Normal", "Inverted", "GND"}
  T85 = typedef "CMI ADS127L21 - Input Impedance.ctl" = enum16{"1M", "1k5"}
  T86 = typedef "CMI ADS127L21 - EXTOUT Mode.ctl" = enum16{"ADCCLK", "REFCLK", "SMPLCLK", "FIRST"}
  T87 = typedef "CMI ADS127L21 - EXTOUT Polarity.ctl" = enum16{"NORM", "INV"}
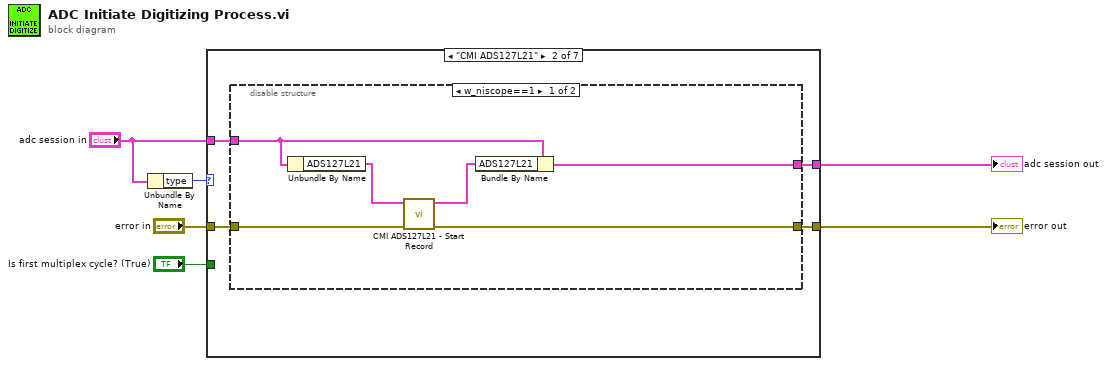
[diagram p0: block diagram]
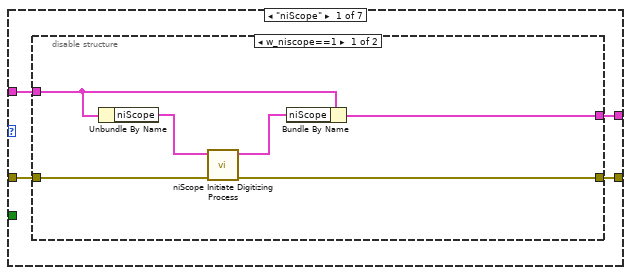
[diagram p2: hidden frame]
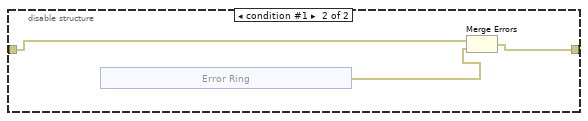
[diagram p3: hidden frame]
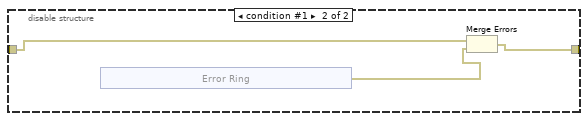
[diagram p4: hidden frame]
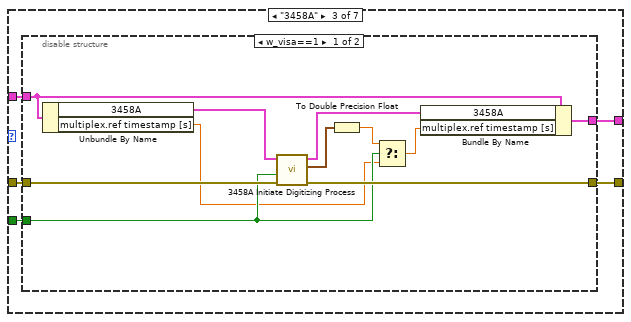
[diagram p5: hidden frame]
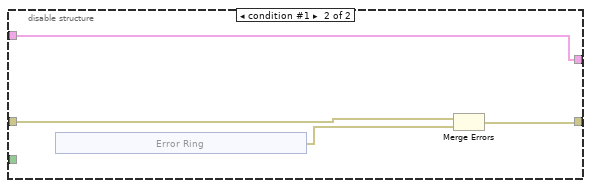
[diagram p6: hidden frame]
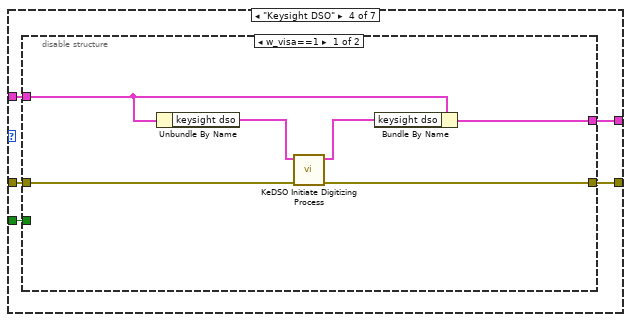
[diagram p7: hidden frame]
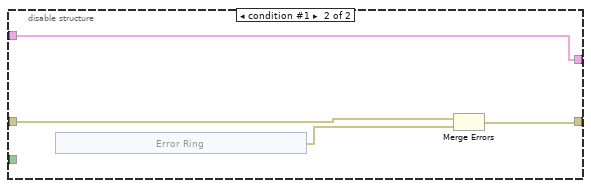
[diagram p8: hidden frame]
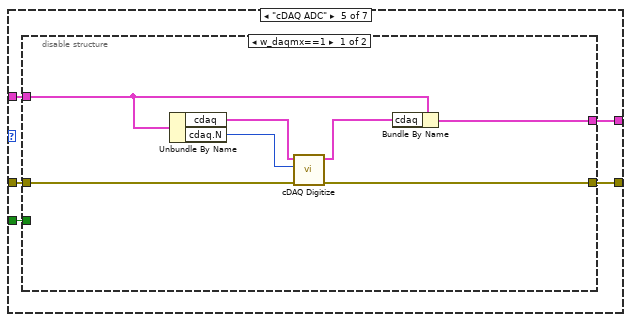
[diagram p9: hidden frame]
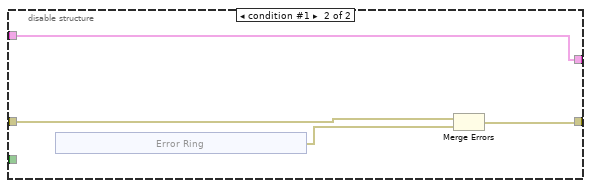
[diagram p10: hidden frame]
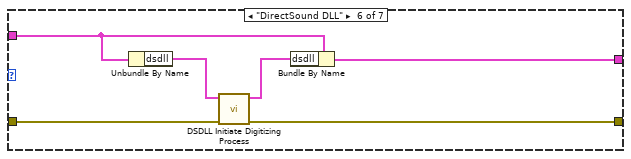
[diagram p11: hidden frame]
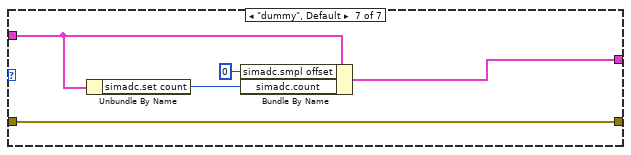
[diagram p12: hidden frame]
diagram:
  n1 = Unbundle By Name("adc session in") -> ("type"=w6:T56)
  n2 = case shown="\"CMI ADS127L21\"" w6 {
    tunnel: "error in" -> [w10 w28 w47 w72 w92 w114 w119]
    tunnel: "adc session in" -> [w9 w27 w46 w71 w91 w112 w117]
    tunnel: [w8 w26 w45 w70 w90 w111 w118] -> w3
    tunnel: [w7 w25 w44 w69 w89 w110 w119] -> w2
    tunnel: "Is first multiplex cycle? (True)" -> [_ _ w43 w68 w88 _ _]
    frame "niScope" {
      n3 = disable-structure shown="w_niscope==1" {
        disable-tunnel: w10 -> [w16 w19]
        disable-tunnel: w9 -> [w14 _]
        disable-tunnel: [w12 _] -> w8
        disable-tunnel: [w11 w18] -> w7
        frame condition #0 (active) {
          n4 = Unbundle By Name(w14) -> ("niScope"=w15:T2)
          n5 = call "niScope Initiate Digitizing Process.vi"("error in"=w16, "niScope in"=w15) -> ("error out"=w11:errorcluster, "niScope out"=w13:T2)  [unwired: 8 in]
          n6 = Bundle By Name(cluster=w14, "niScope"=w13) -> (w12:T1)
        }
        frame condition #1 {
          n7 = xnode "Error Ring"() -> ("error out"=w17:errorcluster)
          n8 = Merge Errors(w19, w17) -> (w18:errorcluster)
        }
      }
    }
    frame "CMI ADS127L21" {
      n9 = disable-structure shown="w_niscope==1" {
        disable-tunnel: w28 -> [w32 w37]
        disable-tunnel: w27 -> [w34 _]
        disable-tunnel: [w33 _] -> w26
        disable-tunnel: [w31 w36] -> w25
        frame condition #0 (active) {
          n10 = Unbundle By Name(w34) -> ("ADS127L21"=w30:T81)
          n11 = call "CMI ADS127L21 - Start Record.vi"("error in (no error)"=w32, "session in"=w30) -> ("error out"=w31:errorcluster, "session out"=w29:T81)  [unwired: 8 in]
          n12 = Bundle By Name(cluster=w34, "ADS127L21"=w29) -> (w33:T1)
        }
        frame condition #1 {
          n13 = xnode "Error Ring"() -> ("error out"=w35:errorcluster)
          n14 = Merge Errors(w37, w35) -> (w36:errorcluster)
        }
      }
    }
    frame "3458A" {
      n15 = disable-structure shown="w_visa==1" {
        disable-tunnel: w47 -> [w58 w61]
        disable-tunnel: w46 -> [w56 w59]
        disable-tunnel: [w55 w59] -> w45
        disable-tunnel: [w54 w60] -> w44
        disable-tunnel: w43 -> [w50 _]
        frame condition #0 (active) {
          n16 = Unbundle By Name(w56) -> ("3458A"=w53:T13, "multiplex.ref timestamp [s]"=w48:dbl)
          n17 = call "3458A Initiate Digitizing Process.vi"("error in"=w58, "Is first multiplex cycle? (True)"=w50, "session in"=w53) -> ("error out"=w54:errorcluster, "initiation timestamp"=w52:timestamp, "session out"=w57:T13)  [unwired: 6 in]
          n18 = To Double Precision Float(number=w52) -> (double precision float=w49:dbl)
          n19 = Select(t=w49, s=w50, f=w48) -> (s? t:f=w51:dbl)
          n20 = Bundle By Name(cluster=w56, "3458A"=w57, "multiplex.ref timestamp [s]"=w51) -> (w55:T1)
        }
        frame condition #1 {
          n21 = xnode "Error Ring"() -> ("error out"=w62:errorcluster)
          n22 = Merge Errors(w61, w62) -> (w60:errorcluster)
        }
      }
    }
    frame "Keysight DSO" {
      n23 = disable-structure shown="w_visa==1" {
        disable-tunnel: w72 -> [w78 w81]
        disable-tunnel: w71 -> [w76 w79]
        disable-tunnel: [w75 w79] -> w70
        disable-tunnel: [w74 w80] -> w69
        disable-tunnel: w68 -> [_ _]
        frame condition #0 (active) {
          n24 = Unbundle By Name(w76) -> ("keysight dso"=w73:T72)
          n25 = call "KeDSO Initiate Digitizing Process.vi"("error in"=w78, "keysight dso"=w73) -> ("error out"=w74:errorcluster, "keysight dso out"=w77:T72)  [unwired: 8 in]
          n26 = Bundle By Name(cluster=w76, "keysight dso"=w77) -> (w75:T1)
        }
        frame condition #1 {
          n27 = xnode "Error Ring"() -> ("error out"=w82:errorcluster)
          n28 = Merge Errors(w81, w82) -> (w80:errorcluster)
        }
      }
    }
    frame "cDAQ ADC" {
      n29 = disable-structure shown="w_daqmx==1" {
        disable-tunnel: w92 -> [w99 w102]
        disable-tunnel: w91 -> [w97 w100]
        disable-tunnel: [w96 w100] -> w90
        disable-tunnel: [w95 w101] -> w89
        disable-tunnel: w88 -> [_ _]
        frame condition #0 (active) {
          n30 = Unbundle By Name(w97) -> ("cdaq"=w94:T78, "cdaq.N"=w93:i32)
          n31 = call "cDAQ Digitize.vi"("error in"=w99, "N"=w93, "cdaq session in"=w94) -> ("error out"=w95:errorcluster, "cdaq session out"=w98:T78)  [unwired: 7 in]
          n32 = Bundle By Name(cluster=w97, "cdaq"=w98) -> (w96:T1)
        }
        frame condition #1 {
          n33 = xnode "Error Ring"() -> ("error out"=w103:errorcluster)
          n34 = Merge Errors(w102, w103) -> (w101:errorcluster)
        }
      }
    }
    frame "DirectSound DLL" {
      n35 = Unbundle By Name(w112) -> ("dsdll"=w109:T52)
      n36 = call "DSDLL Initiate Digitizing Process.vi"("error in"=w114, "dsdll session in"=w109) -> ("error out"=w110:errorcluster, "dsdll session out"=w113:T52)  [unwired: 8 in]
      n37 = Bundle By Name(cluster=w112, "dsdll"=w113) -> (w111:T1)
    }
    frame "dummy", Default {
      n38 = Unbundle By Name(w117) -> ("simadc.set count"=w116:i64)
      n39 = Bundle By Name(cluster=w117, "simadc.smpl offset"=i64 0, "simadc.count"=w116) -> (w118:T1)
    }
  }
  "error out" <- w2
  "adc session out" <- w3
